vi "discrete_transfer_function.run.vi"(4 "reset? (F)":bool, 6 "outut limits (100/0)":cluster{"max_limit":dbl, "min_limit":dbl}={"max_limit"=100.0, "min_limit"=0.0}, 7 "discrete_coefficients":cluster{"b0...bn":dbl[], "a1...an":dbl[]}={"b0...bn"=[0.0, 0.0, 0.0, 0.0], "a1...an"=[0.0, 0.0, 0.0, 0.0]}, 9 "initial_values (0)":cluster{"initial_x":dbl, "initial_y":dbl}, 11 "input":dbl format="%#_13g") -> (3 "output":dbl)   [LabVIEW 2015, in "discrete_control_systems.lvlib"]
doc: "Implements a difference equation of the form:\ny(k) = b0*x(k) + b1*x(k-1) + b2*x(k-2) + b3*x(k-3) + bn*x(k-n) - ( a1*y(k-1) + a2*y(k-2) + a3*y(k-3) + a4*y(k-4) + an*y(k-n) )\n\nThe discrete models are expecting a and b arrays\nthat correspond to a discrete transfer function in the following\nform (from a MATLAB discrete transfer function you may need \nto multiply num and den the by z^-n to get the expected format):\n\n Y(z) b0 + b1*z^-1 + b2*z^-2 + b3*z^-3 + bn*z^-n \nH(z) = ---- = --------------------------------------------------\n X(z) 1 + a1*z^-1 + a2*z^-2 + a3*z^-3 + a4*z^-4 + an*z^-n"
uses:
  discrete_control_systems.lvlib
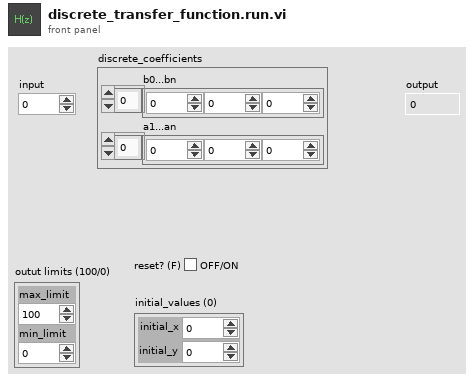
[diagram p1: front panel]
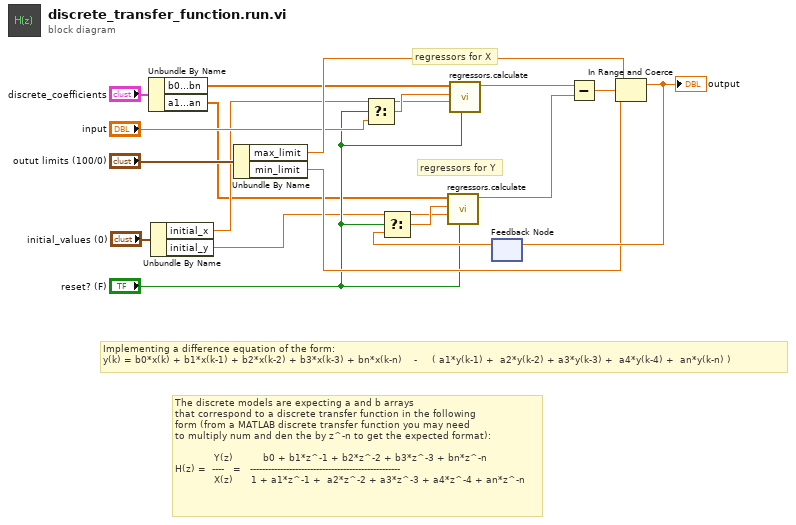
[diagram p0: block diagram]
diagram:
  # "The discrete models are expecting a and b arrays\nthat correspond to a discrete transfer function in the following\nform (from a MATLAB discrete transfer function you may need \nto multiply num and den the by z^-n to get the expected format):\n\n             Y(z)          b0 + b1*z^-1 + b2*z^-2 + b3*z^-3 + bn*z^-n \nH(z) =  ----   =   --------------------------------------------------\n             X(z)      1 + a1*z^-1 +  a2*z^-2 + a3*z^-3 + a4*z^-4 + an*z^-n"
  # "regressors for Y"
  # "regressors for X"
  # "Implementing a difference equation of the form:\ny(k) = b0*x(k) + b1*x(k-1) + b2*x(k-2) + b3*x(k-3) + bn*x(k-n)    -     ( a1*y(k-1) +  a2*y(k-2) + a3*y(k-3) +  a4*y(k-4) +  an*y(k-n) )"
  n1 = Unbundle By Name("discrete_coefficients") -> ("b0...bn"=w2:dbl[], "a1...an"=w1:dbl[])
  n2 = Unbundle By Name("initial_values (0)") -> ("initial_x"=w4:dbl, "initial_y"=w5:dbl)
  n3 = Unbundle By Name("outut limits (100/0)") -> ("max_limit"=w13:dbl, "min_limit"=w12:dbl)
  n4 = Select(t=w4, s="reset? (F)", f="input") -> (s? t:f=w7:dbl)
  n5 = call "regressors.calculate.vi"("reset? (F)"="reset? (F)", "initial_value (0)"=w4, "variable v(k)"=w7, "b0...bn"=w2) -> ("result r(k)"=w18:dbl)  [unwired: 7 in]
  n6 = feedback #1() -> (w11:dbl)  [unwired: 1 in]
  n7 = Select(t=w5, s="reset? (F)", f=w11) -> (s? t:f=w10:dbl)
  n8 = call "regressors.calculate.vi"("reset? (F)"="reset? (F)", "initial_value (0)"=w5, "variable v(k)"=w10, "b0...bn"=w1) -> ("result r(k)"=w17:dbl)  [unwired: 7 in]
  n9 = Subtract(x=w18, y=w17) -> (x-y=w16:dbl)
  n10 = In Range and Coerce(upper limit=w13, x=w16, lower limit=w12) -> (coerced(x)=w15:dbl)  [unwired: 1 out]
  "output" <- w15
  n11 = feedback-in #1(w15) -> ()
